vi "Add Calibration Data.vi"(9 "[TargetLoads]":dbl[](array[numeric])=[0.0, 5.0, 10.0, 20.0, 40.0, 80.0, 160.0], 10 "[A/Ds]":dbl[][](array[numeric])=[[43024.0, 42967.0, 42245.0, 42827.0, 41703.0, 41654.0, 42456.0, 22388.0], [43024.32385392111, 42968.22385392111, 42246.557187254446, 42828.82385392111, 41704.890520587775, 41655.22385392111, 42457.433333333334, 22388.866666666665], [43027.14929239547, 42969.4826257288, 42247.8826257288, 42846.21595906214, 41708.74929239547, 41663.74929239547, 42460.0, 22251.933333333334], [43027.66990857269, 42970.769908572685, 42249.43657523936, 42874.86990857269, 41710.50324190602, 41675.36990857269, 42461.1, 22495.466666666667], [43033.92365817902, 42978.55699151235, 42256.05699151235, 42943.42365817902, 41719.22365817902, 41706.32365817902, 42468.26666666667, 22285.6], [43040.417582664326, 42984.75091599766, 42262.917582664326, 43064.684249330996, 41735.81758266433, 41750.917582664326, 42476.86666666667, 22276.6]], 11 "[Gauge Loads]":dbl[](array[numeric])=[4.85, 10.15, 20.3, 40.2, 78.35]) -> (3 "[CalData]":u8[][](array[numeric]) format="%02x")   [LabVIEW 2013]
uses:
  <vilib>/gmath/NI_Gmath.lvlib
panel:
  out "unsigned 16bit integer":u16[][](array[numeric])
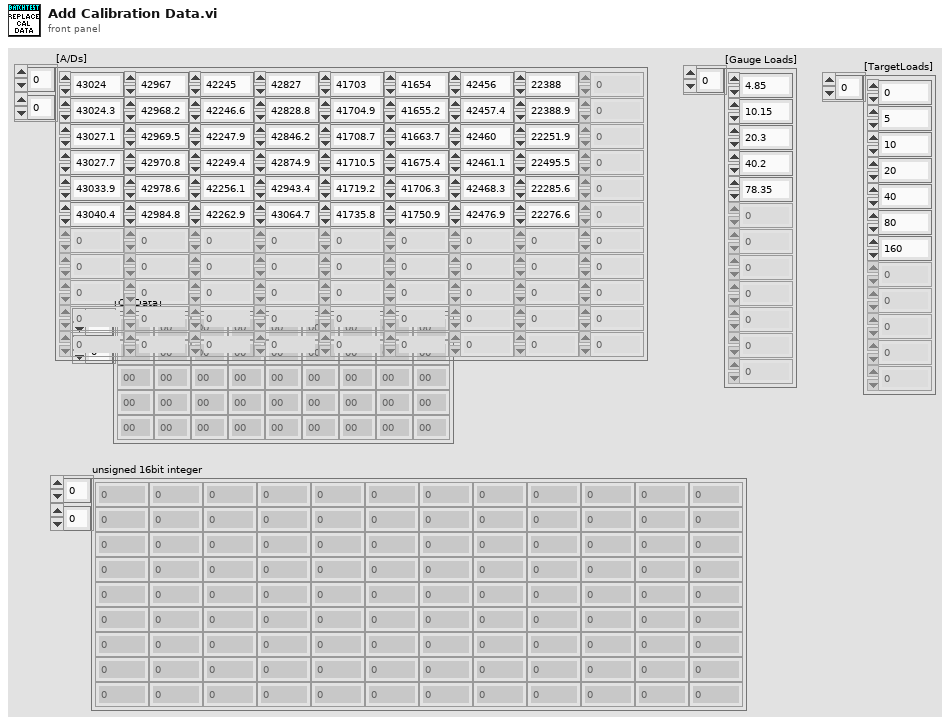
[diagram p1: front panel]
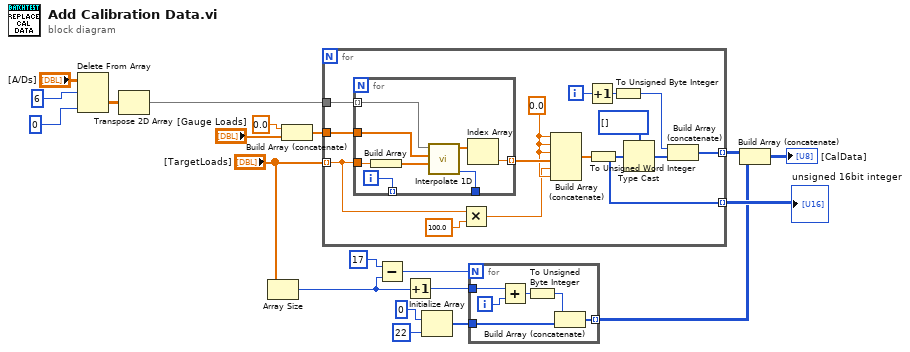
[diagram p0: block diagram]
diagram:
  n1 = Delete From Array(array="[A/Ds]", length=6, index (col)=0 ("disabled index (col)")) -> (deleted portion=w2:dbl[][])  [unwired: 1 in, 1 out]
  n2 = Transpose 2D Array(2D array=w2) -> (transposed array=w1:dbl[][])
  n3 = Array Size(array="[TargetLoads]") -> (size(s)=w6:i32)
  n4 = Build Array (concatenate)(0.0 ("Numeric"), "[Gauge Loads]") -> (w3:dbl[])
  n5 = for {
    tunnel: "[TargetLoads]" -> [w31] mode=indexing
    tunnel: w1 -> [w35]
    tunnel: w3 -> [w34]
    tunnel: [w23] -> w15 mode=indexing
    tunnel: [w21] -> w16 mode=indexing
    i -> [w25]
    w30 = 0.0 ("Numeric")
    n6 = for {
      tunnel: w34 -> [w41]
      tunnel: w35 -> [w40] mode=indexing
      tunnel: w31 -> [w43]
      tunnel: [w38] -> w33 mode=indexing
      tunnel: [w37] -> _
      tunnel: [w36] -> _ mode=indexing
      i -> [w36]
      n7 = Build Array(w43) -> (w42:dbl[])
      n8 = call <vilib>:"Interpolate 1D.vi"("xi"=w42, "X"=w41, "Y"=w40) -> ("error"=w37:i32, "yi"=w39:dbl[])  [unwired: 6 in, 1 out]
      n9 = Index Array(array=w39) -> (element=w38:dbl)  [unwired: 1 in]
    }
    n10 = Multiply(x=w31, y=100.0) -> (x*y=w29:dbl)
    n11 = Build Array (concatenate)(w30, w30, w30, w33, w29, w30) -> (w32:dbl[])
    n12 = Increment(x=w25) -> (x+1=w24:i32)
    n13 = To Unsigned Word Integer(number=w32) -> (unsigned 16bit integer=w21:u16[])
    n14 = To Unsigned Byte Integer(number=w24) -> (unsigned 8bit integer=w22:u8)
    n15 = Type Cast(type=u8[] [] ("unsigned 16bit integer"), x=w21) -> (*(type *) &x=w26:u8[])
    n16 = Build Array (concatenate)(w22, w26) -> (w23:u8[])
  }
  "unsigned 16bit integer" <- w16
  n17 = Subtract(x=17 ("dimension size"), y=w6) -> (x-y=w7:i32)
  n18 = Increment(x=w6) -> (x+1=w5:i32)
  n19 = Initialize Array(u8 0 ("Numeric"), 22 ("dimension size")) -> (w9:u8[])
  n20 = for {
    N: w7 -> [_]
    tunnel: w5 -> [w49]
    tunnel: w9 -> [w48]
    tunnel: [w44] -> w8 mode=indexing
    i -> [w46]
    n21 = Add(x=w49, y=w46) -> (x+y=w47:i32)
    n22 = To Unsigned Byte Integer(number=w47) -> (unsigned 8bit integer=w45:u8)
    n23 = Build Array (concatenate)(w45, w48) -> (w44:u8[])
  }
  n24 = Build Array (concatenate)(w15, w8) -> (→"[CalData]":u8[][])
